vi "Beam Crack Detection.vi"() -> ()   [LabVIEW 2023]
doc: "This example shows the application of computing the bispectrum of a signal to detect cracks of a beam.\n\nDamage detection by means of nondestructive testing is important in ensuring the integrity of machine elements and structures. Cracks of a structure usually generate nonlinear modes. Bispectrum is a useful tool for non-Gaussian signal processing and nonlinearity detection. This example computes both the traditional power spectral density (PSD) and the bispectrum of vibration signals acquired by accelerometers on a normal beam and a cracked beam. From the PSDs of the vibration signals, you hardly can find differences between the normal beam and the cracked beam. From the bispectra of the vibration signals, the cracked beam has significant coupling frequencies. These coupling frequencies indicate system nonlinearities in the cracked beam.\n\nThis example uses the TSA Periodogram VI to compute the traditional PSDs and uses the TSA Bispectrum VI to compute the bispectra of vibration signals from the normal beam and the cracked beam.\n\n<b>Instructions:</b>\n1) Run this VI.\n2) Compare the PSD of the normal beam and cracked beam.\n3) Compare the bispectrum of the normal beam and cracked beam."
uses:
  <vilib>/Native 3D Graph/xcontrol/3DPC_SurfacePlot.xctl
  <vilib>/addons/Time Series Analysis/Utilities.llb/TSA Data.ctl
  <vilib>/addons/Time Series Analysis/Correlation and Spectral Analysis.llb/TSA Periodogram (Waveform).vi
  <vilib>/addons/Time Series Analysis/Correlation and Spectral Analysis.llb/TSA Bispectrum (Waveform).vi
  <vilib>/addons/_Advanced Signal Processing/NI_AdvSigProcTSA.lvlib
panel:
  in  "averaging parameters":T1={"averaging mode"=0, "weighting mode"=0, "number of averages"=10} {"number of averages" min=1; "weighting mode" items=["Linear", "Exponential"]; "averaging mode" items=["No Averaging", "Vector Averaging", "RMS Averaging", "Peak Hold"]}
  in  "Window info":T2={"Window"=1, "Length"=128, "Overlap (%)"=50.0} {"Window" items=["None ", "Hanning", "Hamming", "Blackman-Harris", "Exact Blackman", "Blackman", "Flat Top", "4 Term B-Harris ", "7 Term B-Harris", "Low Sidelobe"]}
  in  "Frequency bins":i32=256
  out "Bispectrum  (Cracked Beam)":refnum<class "Base Datatype.lvclass">[](xcontrol)
  out "Bispectrum  (Normal Beam)":refnum<class "Base Datatype.lvclass">[](xcontrol)
  out "PSD of Vibration Signal":cluster{"f0":dbl, "df":dbl, dbl[][]}(graph)
  # "Overview: Shows the application of computing the bispectrum of a signal to detect cracks of a beam.\nRequirements: LabVIEW Full Development System, Advanced Signal Processing Toolkit\nInstructions: \n1. Run this VI.\n2. Compare the PSD of the normal beam and cracked beam.\n3. Compare the bispectrum of the normal beam and cracked beam."
  # "Bispectrum Settings"
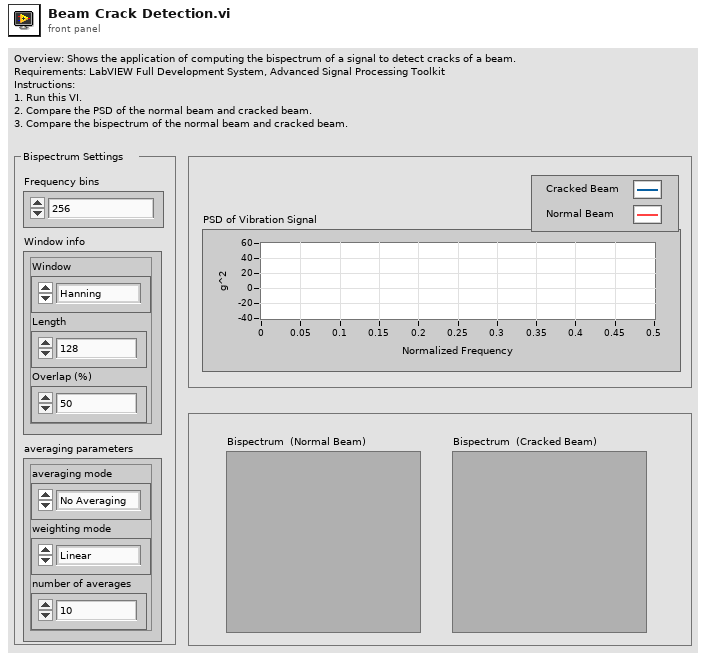
[diagram p1: front panel]
types:
  T1 = cluster{"averaging mode":u16, "weighting mode":u16, "number of averages":u32}
  T2 = cluster{"Window":u16, "Length":i32, "Overlap (%)":dbl}
  T3 = typedef "NI_AdvSigProcTSA.lvlib/TSA Data.ctl" = u16
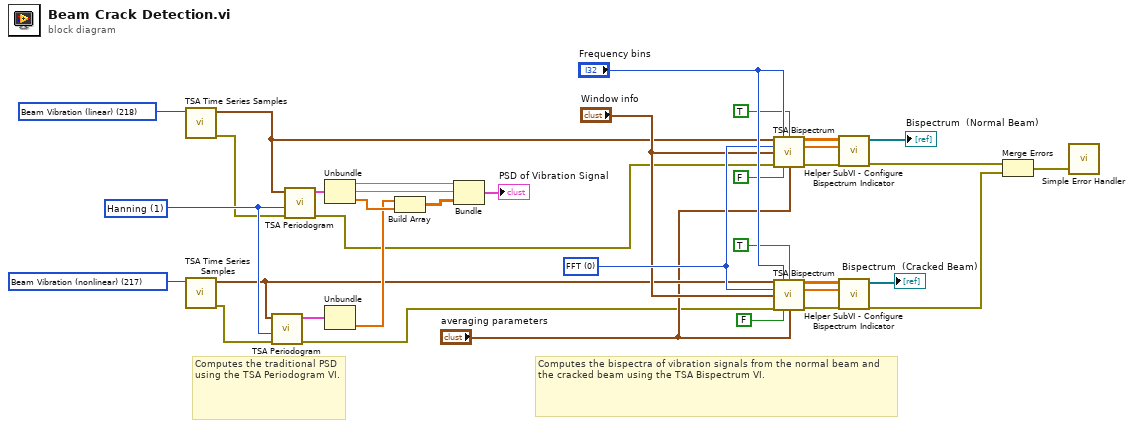
[diagram p0: block diagram]
diagram:
  w20 = T3 217 items=["Kobe Earthquake"=201, "EEG"=210, "Bearing Vibration (simulated)"=211, "Period Product Sales"=214, "Beam Vibration (nonlinear)"=217, "Beam Vibration (linear)"=218, "Signal With Echo"=219, "Engine Knocking"=220, "Power Line"=221, "-"=200, "Beam Deflections (multivariate)"=207, "Structure Vibration (multivariate)"=208, "Human MEG (multivariate)"=222] ("data")
  w21 = T3 218 items=["Kobe Earthquake"=201, "EEG"=210, "Bearing Vibration (simulated)"=211, "Period Product Sales"=214, "Beam Vibration (nonlinear)"=217, "Beam Vibration (linear)"=218, "Signal With Echo"=219, "Engine Knocking"=220, "Power Line"=221, "-"=200, "Beam Deflections (multivariate)"=207, "Structure Vibration (multivariate)"=208, "Human MEG (multivariate)"=222] ("data")
  w24 = u16 1 items=["None ", "Hanning", "Hamming", "Blackman-Harris", "Exact Blackman", "Blackman", "Flat Top", "4 Term B-Harris ", "7 Term B-Harris", "Low Sidelobe"] ("window")
  w28 = u16 0 items=["FFT", "AR Model"] ("method")
  # "Computes the bispectra of vibration signals from the normal beam and the cracked beam using the TSA Bispectrum VI."
  # "Computes the traditional PSD using the TSA Periodogram VI."
  n1 = call <vilib>:"TSA Time Series Samples.vi"("data"=w21) -> ("error out"=w8:errorcluster, "univariate time series"=w23:waveform(dbl))  [unwired: 1 in, 8 out]
  n2 = call <vilib>:"TSA Time Series Samples.vi"("data"=w20) -> ("error out"=w3:errorcluster, "univariate time series"=w22:waveform(dbl))  [unwired: 1 in, 8 out]
  n3 = call-poly <vilib>:"TSA Periodogram.vi"("error in (no error)"=w3, "window"=w24, "Xt"=w22) -> ("error out"=w7:errorcluster, "PSD"=w35:cluster{"f0":dbl, "df":dbl, "S(f)":dbl[]})  [unwired: 2 in, 5 out]
  n4 = call-poly <vilib>:"TSA Periodogram.vi"("error in (no error)"=w8, "window"=w24, "Xt"=w23) -> ("error out"=w9:errorcluster, "PSD"=w36:cluster{"f0":dbl, "df":dbl, "S(f)":dbl[]})  [unwired: 2 in, 5 out]
  n5 = Unbundle(w36) -> ("f0"=w34:dbl, "df"=w33:dbl, "S(f)"=w26:dbl[])
  n6 = Unbundle(w35) -> ("S(f)"=w25:dbl[])  [unwired: 2 out]
  n7 = Build Array(w25, w26) -> (w31:dbl[][])
  n8 = Bundle("f0"=w34, "df"=w33, w31) -> (→"PSD of Vibration Signal":cluster{"f0":dbl, "df":dbl, dbl[][]})  [unwired: 1 out]
  n9 = call-poly <vilib>:"TSA Bispectrum.vi"("Xt"=w23, "frequency bins"="Frequency bins", "initialize? (F)"=TRUE, "method"=w28, "window info"="Window info", "error in (no error)"=w9, "dB on? (T)"=FALSE, "averaging parameters"="averaging parameters") -> ("S(f,f)"=w16:dbl[][], "freq bins"=w15:dbl[], "error out"=w12:errorcluster)  [unwired: 3 in, 2 out]
  n10 = call-poly <vilib>:"TSA Bispectrum.vi"("Xt"=w22, "frequency bins"="Frequency bins", "initialize? (F)"=TRUE, "method"=w28, "window info"="Window info", "error in (no error)"=w7, "dB on? (T)"=FALSE ("dB On? (T)"), "averaging parameters"="averaging parameters") -> ("S(f,f)"=w14:dbl[][], "freq bins"=w13:dbl[], "error out"=w11:errorcluster)  [unwired: 3 in, 2 out]
  n11 = call "Helper SubVI - Configure Bispectrum Indicator.vi"("error in (no error)"=w12, "frequency bins"=w15, "S(f,f)"=w16) -> ("error out"=w6:errorcluster, "bispectrum  indicator"=→"Bispectrum  (Normal Beam)":refnum<class "Base Datatype.lvclass">[])  [unwired: 7 in]
  n12 = call "Helper SubVI - Configure Bispectrum Indicator.vi"("error in (no error)"=w11, "frequency bins"=w13, "S(f,f)"=w14) -> ("error out"=w5:errorcluster, "bispectrum  indicator"=→"Bispectrum  (Cracked Beam)":refnum<class "Base Datatype.lvclass">[])  [unwired: 7 in]
  n13 = Merge Errors(w6, w5) -> (w4:errorcluster)
  n14 = call <vilib>:"Simple Error Handler.vi"("error in (no error)"=w4) -> ()  [unwired: 4 in, 5 out]
